vi "1-Tap 8-Bit Camera with Centroid (FPGA).vi"() -> ()   [LabVIEW 2012]
doc: "This is the FPGA VI for the 1-Tap 8-Bit Camera with Centroid example. This example demonstrates how to perform image processing operations on the FPGA in real time. This example performs an image thresholding operation, which can be controlled via the host VI, followed by a centroid computation. The processed images and centroid coordinates are then transfered to the host, using DMA, so that they can be displayed.\n\nAdditionally, the example demonstrates the serial server, which allows third-party camera configuration utilities to communicate with the camera using the Camera Link serial interface while this VI is running."
uses:
  Common/CL Signal Mapping.ctl
  Common/CL Configuration.ctl
  <vilib>/Platform/TimedLoop/XDataNode/timing_clust.ctl
  <vilib>/Platform/TimedLoop/XDataNode/nitl_modes.ctl
  <vilib>/Platform/TimedLoop/XDataNode/wakeup.ctl
  <vilib>/rvi/eio/common/nirviEmuTemplateMethod_errors.vi
  <vilib>/rvi/Emulation/niFpgaSctlEmulationRegisterWithScheduler.vi
  <vilib>/rvi/Emulation/niFpgaSctlEmulationScheduler.vi
  Common/CL Data to Pixels/1 Tap 8-Bit.vi
  <vilib>/rvi/interface/RandomDataEmulation/nirviRandomDataFPGAFIFO.vi
  <vilib>/rvi/interface/RandomDataEmulation/niFpgaRandomDataHandleErrors.vi
  <vilib>/rvi/Emulation/niFpgaSctlEmulationGlobalWrite.vi
  <vilib>/Platform/TimedLoop/XDataNode/XDataNode.xnode
  <vilib>/eio/EIONode/EIONode.xnode
  <vilib>/rvi/DataTransferAndStorage/Container/XNode/niFpgaContainer.xnode
  <vilib>/rvi/interface/RandomDataEmulation/nirviRandomDataFpgaReadWriteTemplate.vi
  <vilib>/Platform/TimedLoop/XDataNode/XDNodeRunTimeDep.lvlib
panel:
  in  "CL Config.Configuration":T1
  in  "CL Config.Signal Mapping":T2
  in  "CL Config.Line Scan":bool
  in  "CL Config.DVAL Active High":bool=TRUE
  in  "CL Config.LVAL Active High":bool=TRUE
  in  "CL Config.FVAL Active High":bool=TRUE
  in  "CL Config.Spare Active High":bool=TRUE
  in  "Threshold.Invert":bool
  in  "Threshold.Upper Limit":u8=127
  in  "Threshold.Lower Limit":u8
  in  "Threshold.Replace":bool
  in  "Threshold.Replacement":u8=255
  in  "Centroid.Image Width":u16=640
  in  "Centroid.Image Height":u16=480
  in  "Acq Control.Line Scan Height":u32
  in  "Acq Control.Frames To Acq":u32
  in  "Acq Control.Acquire":bool
  in  "Acq Control.Cancel Acq":bool
  in  "Acq Control.Ignore DVAL":bool
  in  "Acq Control.Initialize":bool
  out "Acq Status.Acq In Progress":bool
  out "Acq Status.Clocks Per Line":u32
  out "Acq Status.Frames Acq'd":u32
  out "Acq Status.Lines Per Frame":u32
  out "Acq Status.DMA Write Timeout":bool
  out "Acq Status.Initialized":bool
  in  "UART.Baud Rate":u8
  in  "UART.Transmit":bool
  in  "UART.Tx Data":u8[](array[numeric])=[0, 0, 0, 0, 0, 0, 0, 0, 0, 0] format="%02x"
  in  "UART.Set Baud Rate":bool
  in  "UART.Byte Mode":bool=TRUE
  out "UART.Rx Ready":bool
  out "UART.Break Indicator":bool
  out "UART.Framing Error":bool
  out "UART.Overrun Error":bool
  out "UART.Tx Ready":bool
  out "UART.Rx Data":u8 format="%02x"
  in  "UART.Receive":bool
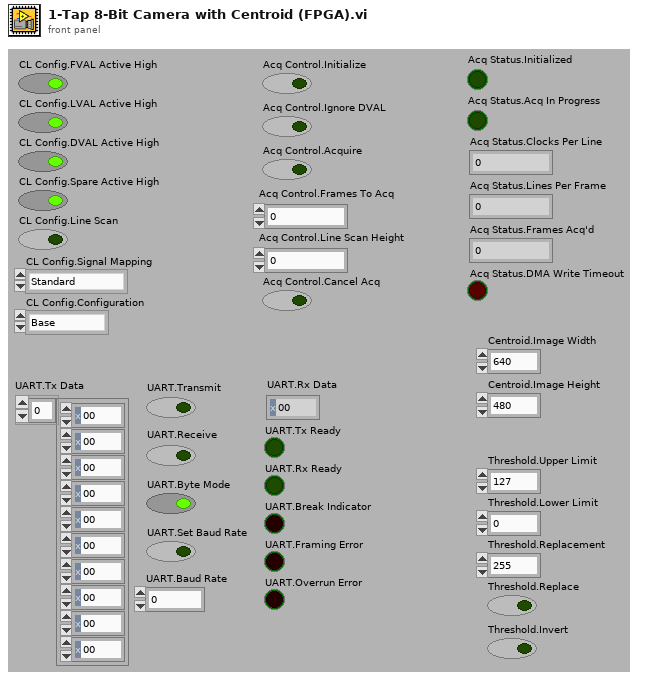
[diagram p1: front panel]
types:
  T1 = typedef "CL Configuration.ctl" = enum8{"Base", "Medium", "Full"}
  T2 = typedef "CL Signal Mapping.ctl" = enum8{"Standard", "Basler 10-tap", "Vosskühler 10-tap"}
  T3 = typedef "XDNodeRunTimeDep.lvlib/timing_clust.ctl" = cluster{"Expected End [f-1]":u64, "Actual End [f-1]":u64, "Finished Late? [f-1]":bool, "Expected End [i-1]":u64, "Actual End [i-1]":u64, "Finished Late? [i-1]":bool, "Expected Start [i]":u64, "Actual Start [i]":u64, "Expected Start [f]":u64, "Actual Start [f]":u64, "Source Name":string, "Structure Name":string, "Period":i64, "Deadline":i64, "Offset":i64, "Start":i64, "Priority":i32, "Timeout":i32, "Mode":T4, "Wakeup Reason":T5, "Error":errorcluster, "Source Type":string, "Secondary Source Type":string, "Global End Time":u64, "Global Start Time":u64, "Frame Duration":u64, "Iteration Duration":u64, "Assigned CPU":i32, "I/O Scan Engine Mode":u32}
  T4 = typedef "XDNodeRunTimeDep.lvlib/nitl_modes.ctl" = enum32{"No Change", "Process missed periods, maintain original phase", "Discard missed periods, maintain original phase", "Process missed periods, ignore original phase", "Discard missed periods, ignore original phase"}
  T5 = typedef "XDNodeRunTimeDep.lvlib/wakeup.ctl" = enum32{"Normal", "Aborted", "Asynchronous wakeup", "Timing source error", "Timed loop error", "Timeout"}
  T6 = cluster{"Enables Valid":bool, "Frame Valid":bool, "Line Valid":bool, "Data Valid":bool}
  T7 = cluster{"Tx Data":u8[], "Transmit":bool, "Receive":bool, "Byte Mode":bool, "Set Baud Rate":bool, "Baud Rate":u8}
  T8 = cluster{"Rx Data":u8, "Turn Off Transmit":bool, "Turn Off Receive":bool, "Turn Off Set Baud Rate":bool, "Tx Ready":bool, "Rx Ready":bool, "Break Indicator":bool, "Framing Error":bool, "Overrun Error":bool}
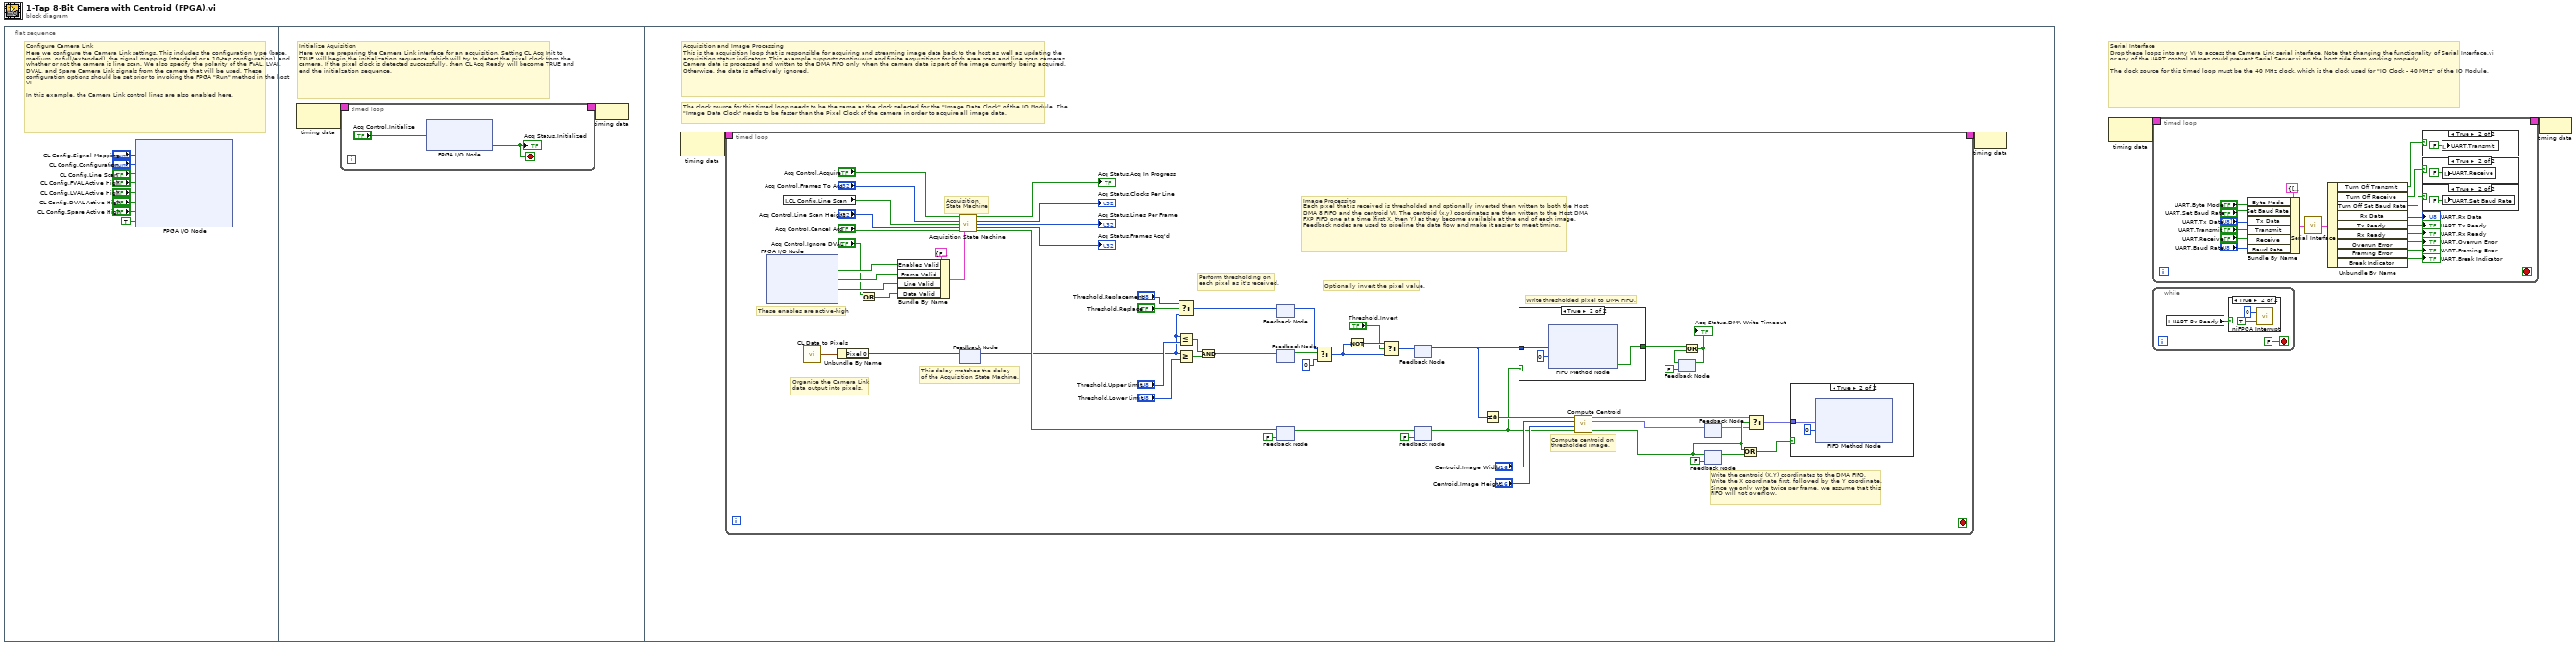
[diagram p0: block diagram]
diagram:
  # "Serial Interface\nDrop these loops into any VI to access the Camera Link serial interface. Note that changing the functionality of Serial Interface.vi or any of the UART control names could prevent Serial Server.vi on the host side from working properly.\n\nThe clock source for this timed loop must be the 40 MHz clock, which is the clock used for \"IO Clock - 40 MHz\" of the IO Module."
  n1 = flat-sequence {
    frame #0 {
      # "Configure Camera Link\nHere we configure the Camera Link settings. This includes the configuration type (base, medium, or full/extended), the signal mapping (standard or a 10-tap configuration), and whether or not the camera is line scan. We also specify the polarity of the FVAL, LVAL, DVAL, and Spare Camera Link signals from the camera that will be used. These configuration options should be set prior to invoking the FPGA \"Run\" method in the host VI.\n\nIn this example, the Camera Link control lines are also enabled here."
      n2 = xnode "FPGA I/O Node"("CL Set Signal Mapping"="CL Config.Signal Mapping", "CL Set Configuration"="CL Config.Configuration", "CL Set Line Scan"="CL Config.Line Scan", "CL Set FVAL Active High"="CL Config.FVAL Active High", "CL Set LVAL Active High"="CL Config.LVAL Active High", "CL Set DVAL Active High"="CL Config.DVAL Active High", "CL Set Spare Active High"="CL Config.Spare Active High", "CL Control Enable"=TRUE ("IO Module\\CL Control Enable")) -> ()  [unwired: 8 in, 8 out]
    }
    frame #1 {
      # "Initialize Aquisition\nHere we are preparing the Camera Link interface for an acquisition. Setting CL Acq Init to TRUE will begin the initialization sequence, which will try to detect the pixel clock from the camera. If the pixel clock is detected successfully, then CL Acq Ready will become TRUE and end the initialzation sequence."
      n3 = node-c288() -> (w12:T3)  [unwired: 1 out]
      n4 = timed-loop {
        timing: w12 -> [_]
        timing-out: [_] -> w11
        stop <- w13 stop-if-true
        n5 = xnode "FPGA I/O Node"("CL Acq Init"="Acq Control.Initialize") -> ("CL Acq Ready"=w13:bool)  [unwired: 2 in, 2 out]
        "Acq Status.Initialized" <- w13
      }
      n6 = node-c288(w11) -> ()
    }
    frame #2 {
      # "The clock source for this timed loop needs to be the same as the clock selected for the \"Image Data Clock\" of the IO Module. The \"Image Data Clock\" needs to be faster than the Pixel Clock of the camera in order to acquire all image data."
      # "Acquisition and Image Processing\nThis is the acquisition loop that is responsible for acquiring and streaming image data back to the host as well as updating the acquisition status indicators. This example supports continuous and finite acquisitions for both area scan and line scan cameras. Camera data is processed and written to the DMA FIFO only when the camera data is part of the image currently being acquired. Otherwise, the data is effectively ignored."
      n7 = node-c288() -> (w20:T3)  [unwired: 1 in]
      n8 = timed-loop {
        timing: w20 -> [_]
        timing-out: [_] -> w19
        stop <- _ stop-if-true
        # "Optionally invert the pixel value."
        # "Image Processing\nEach pixel that is received is thresholded and optionally inverted then written to both the Host DMA 8 FIFO and the centroid VI. The centroid (x,y) coordinates are then written to the Host DMA FXP FIFO one at a time (first X, then Y) as they become available at the end of each image. Feedback nodes are used to pipeline the data flow and make it easier to meet timing."
        # "Write thresholded pixel to DMA FIFO."
        # "Perform thresholding on\neach pixel as it's received."
        # "Write the centroid (X,Y) coordinates to the DMA FIFO. \nWrite the X coordinate first, followed by the Y coordinate.\nSince we only write twice per frame, we assume that this \nFIFO will not overflow."
        # "Compute centroid on\nthresholded image."
        # "Organize the Camera Link\ndata output into pixels."
        # "These enables are active-high"
        # "This delay matches the delay\nof the Acquisition State Machine."
        # "Acquisition\nState Machine"
        n9 = xnode "FPGA I/O Node"() -> ("CL Output Valid"=w67:bool, "CL Frame Valid"=w66:bool, "CL Line Valid"=w65:bool, "CL Data Valid"=w62:bool)  [unwired: 4 in, 4 out]
        n10 = local read "CL Config.Line Scan"() -> (w59:bool)
        n11 = call-poly "CL Data to Pixels.vi"() -> ("Pixels"=w76:cluster{"Pixel 0":u8})  [unwired: 1 in]
        n12 = Unbundle By Name(w76) -> ("Pixel 0"=w75:u8)
        n13 = Or(x="Acq Control.Ignore DVAL", y=w62) -> (x .or. y?=w61:bool)
        n14 = Bundle By Name(cluster=T6 {"Enables Valid"=FALSE, "Frame Valid"=FALSE, "Line Valid"=FALSE, "Data Valid"=FALSE} ("Enables"), "Enables Valid"=w67, "Frame Valid"=w66, "Line Valid"=w65, "Data Valid"=w61) -> (w64:T6)
        n15 = call "Acquisition State Machine.vi"("Acquire"="Acq Control.Acquire", "Frames to Acquire"="Acq Control.Frames To Acq", "Line Scan"=w59, "Line Scan Height"="Acq Control.Line Scan Height", "Cancel Acq"="Acq Control.Cancel Acq", "Enables"=w64) -> ("Acq In Progress"=→"Acq Status.Acq In Progress":bool, "Num Clocks Per Line"=→"Acq Status.Clocks Per Line":u32, "Num Lines Per Frame"=→"Acq Status.Lines Per Frame":u32, "Num Frames Acq'd"=→"Acq Status.Frames Acq'd":u32, "Capture Cycle"=w30:bool)  [unwired: 4 in, 1 out]
        n16 = feedback-in #1(w75) -> ()
        n17 = feedback #1() -> (w29:u8)  [unwired: 1 in]
        n18 = Select(t="Threshold.Replacement", s="Threshold.Replace", f=w29) -> (s? t:f=w41:u8)
        n19 = Less Or Equal?(x=w29, y="Threshold.Upper Limit") -> (x <= y?=w36:bool)
        n20 = Greater Or Equal?(x=w29, y="Threshold.Lower Limit") -> (x >= y?=w35:bool)
        n21 = And(x=w36, y=w35) -> (x .and. y?=w43:bool)
        n22 = feedback #2() -> (w42:u8)  [unwired: 1 in]
        n23 = feedback-in #2(w41) -> ()
        n24 = feedback #3() -> (w44:bool)  [unwired: 1 in]
        n25 = feedback-in #3(w43) -> ()
        n26 = feedback #4(FALSE ("Capture Cycle")) -> (w46:bool)
        n27 = feedback-in #4(w30) -> ()
        n28 = Select(t=w42, s=w44, f=u8 0) -> (s? t:f=w39:u8)
        n29 = Not(x=w39) -> (.not. x?=w40:u8)
        n30 = Select(t=w40, s="Threshold.Invert", f=w39) -> (s? t:f=w45:u8)
        n31 = feedback #5() -> (w25:u8)  [unwired: 1 in]
        n32 = feedback-in #5(w45) -> ()
        n33 = feedback #6(FALSE ("Capture Cycle")) -> (w21:bool)
        n34 = feedback-in #6(w46) -> ()
        n35 = Not Equal To 0?(x=w25) -> (x != 0?=w22:bool)
        n36 = case shown="True" w21 {
          tunnel: w25 -> [_ w80]
          tunnel: [_ w79] -> w57
          frame False {
          }
          frame True {
            n37 = xnode ("FIFO Method Node")("Element"=w80, "Timeout"=0) -> ("Timed Out?"=w79:bool)  [unwired: 1 in, 1 out]
          }
        }
        n38 = call "Compute Centroid.vi"("Input Valid"=w21, "Image Height"="Centroid.Image Height", "Image Width"="Centroid.Image Width", "Pixel"=w22) -> ("Output valid"=w52:bool, "Y"=w51:fxp<+,32,16>, "X"=w50:fxp<+,32,16>)  [unwired: 5 in]
        n39 = feedback #7(FALSE) -> (w55:bool)
        n40 = Or(x=w57, y=w55) -> (x .or. y?=w54:bool)
        "Acq Status.DMA Write Timeout" <- w54
        n41 = feedback-in #7(w54) -> ()
        n42 = feedback #8() -> (w47:fxp<+,32,16>)  [unwired: 1 in]
        n43 = feedback-in #8(w51) -> ()
        n44 = feedback #9(FALSE ("Output valid")) -> (w48:bool)
        n45 = feedback-in #9(w52) -> ()
        n46 = Or(x=w52, y=w48) -> (x .or. y?=w53:bool)
        n47 = Select(t=w50, s=w52, f=w47) -> (s? t:f=w49:fxp<+,32,16>)
        n48 = case shown="True" w53 {
          tunnel: w49 -> [_ w77]
          frame False {
          }
          frame True {
            n49 = xnode ("FIFO Method Node")("Element"=w77, "Timeout"=0) -> ()  [unwired: 1 in, 2 out]
          }
        }
      }
      n50 = node-c288(w19) -> ()
    }
  }
  n51 = node-c288() -> (w2:T3)  [unwired: 1 out]
  n52 = timed-loop {
    timing: w2 -> [_]
    timing-out: [_] -> w1
    stop <- _ stop-if-true
    n53 = Bundle By Name(cluster=T7 {"Tx Data"=[0, 0, 0, 0, 0, 0, 0, 0, 0, 0], "Transmit"=FALSE, "Receive"=FALSE, "Byte Mode"=TRUE, "Set Baud Rate"=FALSE, "Baud Rate"=0} ("UART Inputs"), "Byte Mode"="UART.Byte Mode", "Set Baud Rate"="UART.Set Baud Rate", "Tx Data"="UART.Tx Data", "Transmit"="UART.Transmit", "Receive"="UART.Receive", "Baud Rate"="UART.Baud Rate") -> (w86:T7)
    n54 = call "Serial Interface.vi"("UART Inputs"=w86) -> ("UART Outputs"=w98:T8)
    n55 = Unbundle By Name(w98) -> ("Turn Off Transmit"=w91:bool, "Turn Off Receive"=w92:bool, "Turn Off Set Baud Rate"=w88:bool, "Rx Data"=→"UART.Rx Data":u8, "Tx Ready"=→"UART.Tx Ready":bool, "Rx Ready"=→"UART.Rx Ready":bool, "Overrun Error"=→"UART.Overrun Error":bool, "Framing Error"=→"UART.Framing Error":bool, "Break Indicator"=→"UART.Break Indicator":bool)
    n56 = case shown="True" w91 {
      frame False {
      }
      frame True {
        n57 = local write "UART.Transmit"(FALSE ("UART.Transmit")) -> ()
      }
    }
    n58 = case shown="True" w92 {
      frame False {
      }
      frame True {
        n59 = local write "UART.Receive"(FALSE ("UART.Receive")) -> ()
      }
    }
    n60 = case shown="True" w88 {
      frame False {
      }
      frame True {
        n61 = local write "UART.Set Baud Rate"(FALSE ("UART.Receive")) -> ()
      }
    }
  }
  n62 = while {
    stop <- FALSE stop-if-true
    n63 = local read "UART.Rx Ready"() -> (w110:bool)
    n64 = case shown="True" w110 {
      frame False {
      }
      frame True {
        n65 = call <vilib>:"niFPGA Interrupt.vi"("Wait Until Cleared (F)"=TRUE ("Wait Until Cleared"), "IRQ Number (0)"=u8 0 ("IRQ Number")) -> ()  [unwired: 1 in]
      }
    }
  }
  n66 = node-c288(w1) -> ()
